vi "TSLIN_Schedule_Table_Display.vi"(8 "错误输入（无错误）":errorcluster, 10 "LIN Scheduling Table Array":T1[](array[typedef]) {"LIN_Transmit"."Channel" items=["CHN1", "CHN2", "CHN3", "CHN4", "CHN5", "CHN6", "CHN7", "CHN8", "CHN9", "CHN10", "CHN11", "CHN12", "CHN13", "CHN14", "CHN15", "CHN16", "CHN17", "CHN18", "CHN19", "CHN20", "CHN21", "CHN22", "CHN23", "CHN24", "CHN25", "CHN26", "CHN27", "CHN28", "CHN29", "CHN30", "CHN31", "CHN32"]; "LIN_Transmit"."ID" format="%.0x"; "LIN_Transmit"."DLC" format="%.0x"; "LIN_Transmit"."Set_node_funtiontype" items=["MasterNode", "SlaveNode", "MonitorNote"]}, 11 "LIN_Data Ref":refnum<vi>) -> (0 "错误输出":errorcluster)   [LabVIEW 2014]
uses:
  Typedef/TSLIN_Transmit.ctl
  Typedef/TSLIN_LIN Schedule_Table.ctl
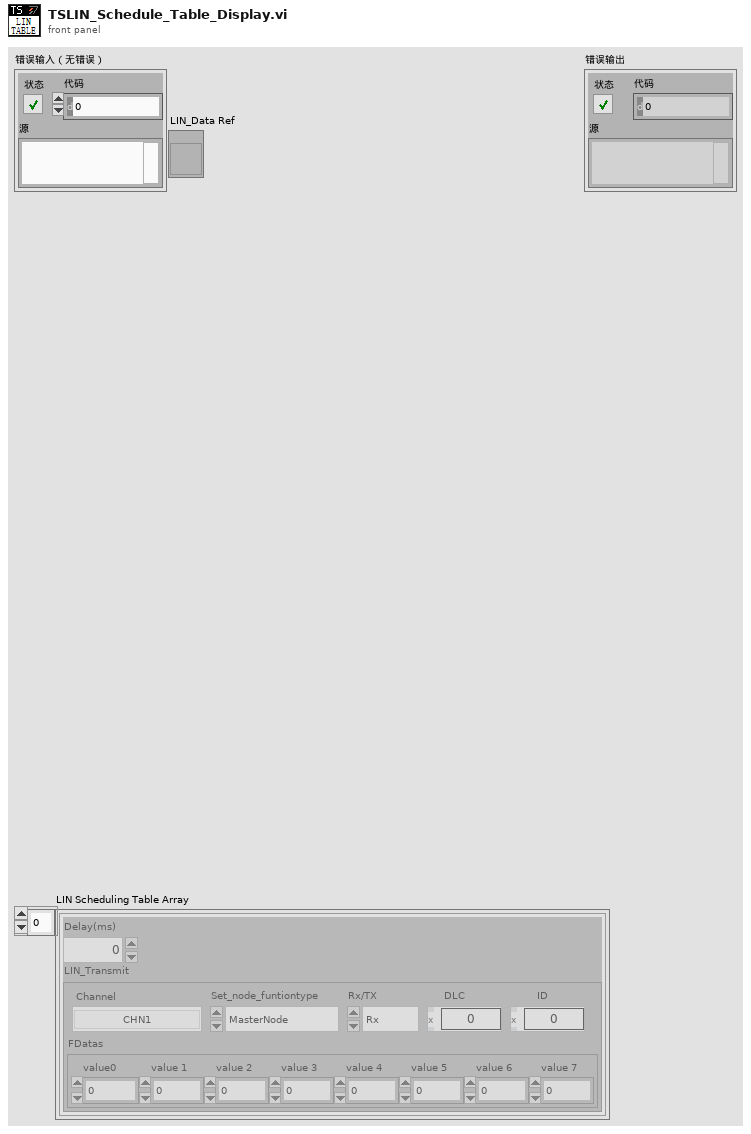
[diagram p1: front panel]
types:
  T1 = typedef "TSLIN_LIN Schedule_Table.ctl" = cluster{"LIN_Transmit":T2, "Delay(ms)":i32}
  T2 = typedef "TSLIN_Transmit.ctl" = cluster{"Channel":i32, "Rx/TX":enum16{"Rx", "Tx"}, "Set_node_funtiontype":i32, "DLC":u32, "ID":u32, "FDatas":cluster{"value0":u8, "value 1":u8, "value 2":u8, "value 3":u8, "value 4":u8, "value 5":u8, "value 6":u8, "value 7":u8}}
  T3 = cluster{"value0":u8, "value 1":u8, "value 2":u8, "value 3":u8, "value 4":u8, "value 5":u8, "value 6":u8, "value 7":u8}
  T4 = typedef "LVRowAndColumnUnsignedTypeDef.ctl" = cluster{"Row":u32, "Column":u32}
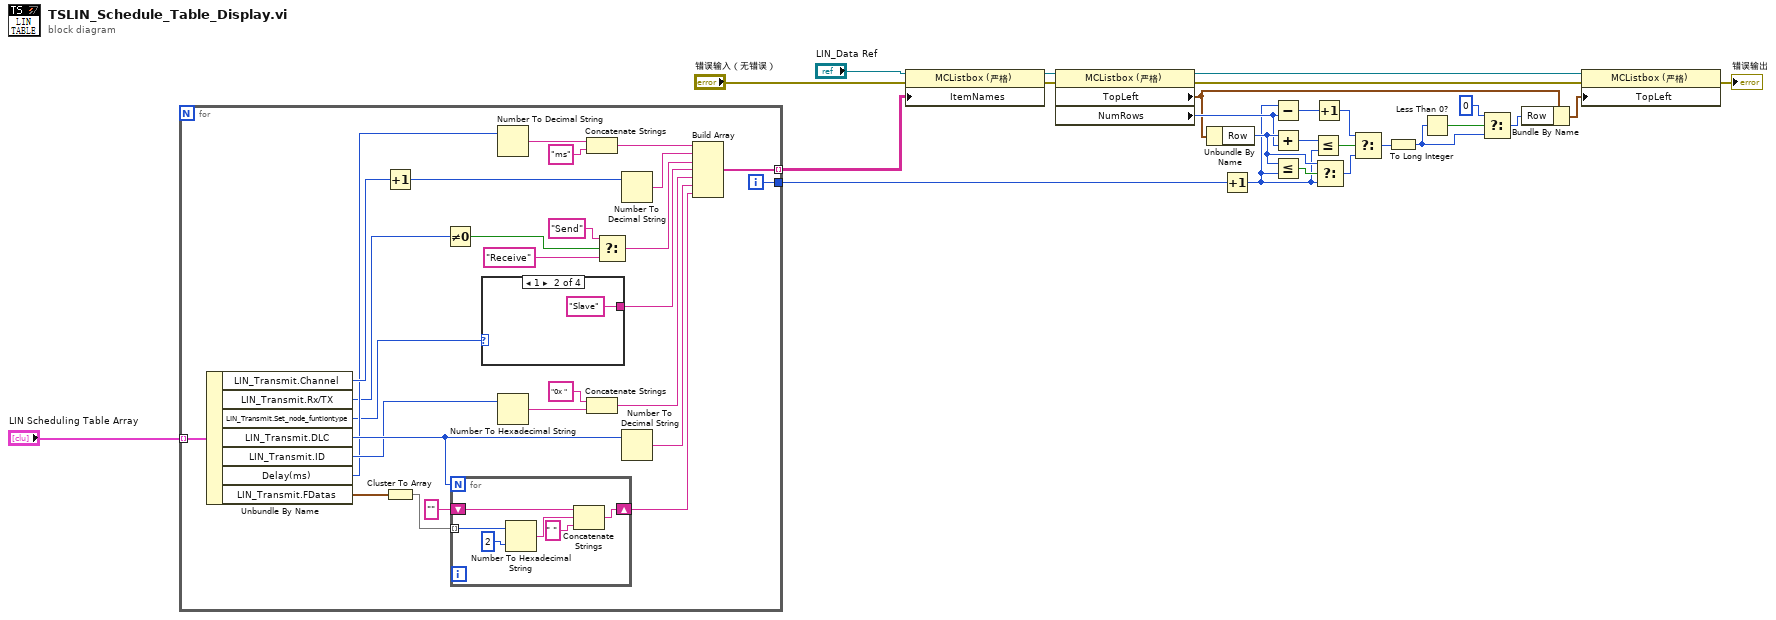
[diagram p0: block diagram]
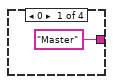
[diagram p2: hidden frame]
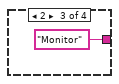
[diagram p3: hidden frame]
diagram:
  n1 = for {
    tunnel: "LIN Scheduling Table Array" -> [w53] mode=indexing
    tunnel: [w41] -> w26 mode=indexing
    tunnel: [w31] -> w2
    i -> [w31]
    n2 = Unbundle By Name(w53) -> ("LIN_Transmit.Channel"=w40:i32, "LIN_Transmit.Rx/TX"=w29:enum16{"Rx", "Tx"}, "LIN_Transmit.Set_node_funtiontype"=w27:i32, "LIN_Transmit.DLC"=w48:u32, "LIN_Transmit.ID"=w32:u32, "Delay(ms)"=w30:i32, "LIN_Transmit.FDatas"=w49:T3)
    n3 = Increment(x=w40) -> (x+1=w39:i32)
    n4 = Cluster To Array(cluster=w49) -> (array=w47:u8[])
    n5 = Not Equal To 0?(x=w29) -> (x != 0?=w28:bool)
    n6 = for {
      N: w48 -> [_]
      tunnel: w47 -> [w59] mode=indexing
      shift-right: [w61] -> w42
      shift-left: "" -> [w62]
      n7 = Number To Hexadecimal String(1:i16 2 ("width (-)"), 2:w59) -> (0:w58:string)
      n8 = Concatenate Strings(w62, w58, " " ("string")) -> (w61:string)
    }
    n9 = case shown="1" w27 {
      tunnel: ["Master" "Slave" "Monitor" _] -> w44
      frame 0 {
      }
      frame 1 {
      }
      frame 2 {
      }
      frame 3, Default {
      }
    }
    n10 = Number To Decimal String(number=w30) -> (decimal integer string=w34:string)  [unwired: 1 in]
    n11 = Number To Hexadecimal String(2:w32) -> (0:w37:string)  [unwired: 1 in]
    n12 = Concatenate Strings(w34, "ms" ("字符串")) -> (w35:string)
    n13 = Concatenate Strings("0x " ("字符串"), w37) -> (w38:string)
    n14 = Select(t="Send", s=w28, f="Receive") -> (s? t:f=w45:string)
    n15 = Number To Decimal String(number=w39) -> (decimal integer string=w46:string)  [unwired: 1 in]
    n16 = Number To Decimal String(number=w48) -> (decimal integer string=w43:string)  [unwired: 1 in]
    n17 = Build Array(w35, w46, w45, w44, w38, w43, w42) -> (w41:string[])
  }
  n18 = property class="MCListbox (严格)"(reference="LIN_Data Ref", error in="错误输入（无错误）", "ItemNames"=w26) -> (reference out=w8:refnum<vi>, error out=w6:errorcluster)
  n19 = property class="MCListbox (严格)"(reference=w8, error in=w6) -> (reference out=w16:refnum<vi>, error out=w5:errorcluster, "TopLeft"=w15:T4, "NumRows"=w23:u32)
  n20 = Unbundle By Name(w15) -> ("Row"=w24:u32)
  n21 = Increment(x=w2) -> (x+1=w21:i32)
  n22 = Subtract(x=w21, y=w23) -> (x-y=w20:u32)
  n23 = Add(x=w24, y=w23) -> (x+y=w22:u32)
  n24 = Less Or Equal?(x=w24, y=w21) -> (x <= y?=w25:bool)
  n25 = Less Or Equal?(x=w22, y=w21) -> (x <= y?=w17:bool)
  n26 = Increment(x=w20) -> (x+1=w18:u32)
  n27 = Select(t=w24, s=w25, f=w21) -> (s? t:f=w19:u32)
  n28 = Select(t=w18, s=w17, f=w19) -> (s? t:f=w14:u32)
  n29 = To Long Integer(number=w14) -> (32bit integer=w12:i32)
  n30 = Less Than 0?(x=w12) -> (x < 0?=w13:bool)
  n31 = Select(t=0, s=w13, f=w12) -> (s? t:f=w11:i32)
  n32 = Bundle By Name(cluster=w15, "Row"=w11) -> (w9:T4)
  n33 = property class="MCListbox (严格)"(reference=w16, error in=w5, "TopLeft"=w9) -> (error out=→"错误输出":errorcluster)  [unwired: 1 out]
